vi "queue packet to transmit.vi"(8 "error in (no error)":errorcluster, 10 "Packet":string, 11 "data passing":T1) -> (0 "error out":errorcluster, 3 "data passing out":T1)   [LabVIEW 2016]
uses:
  data.ctl
  device/device.ctl
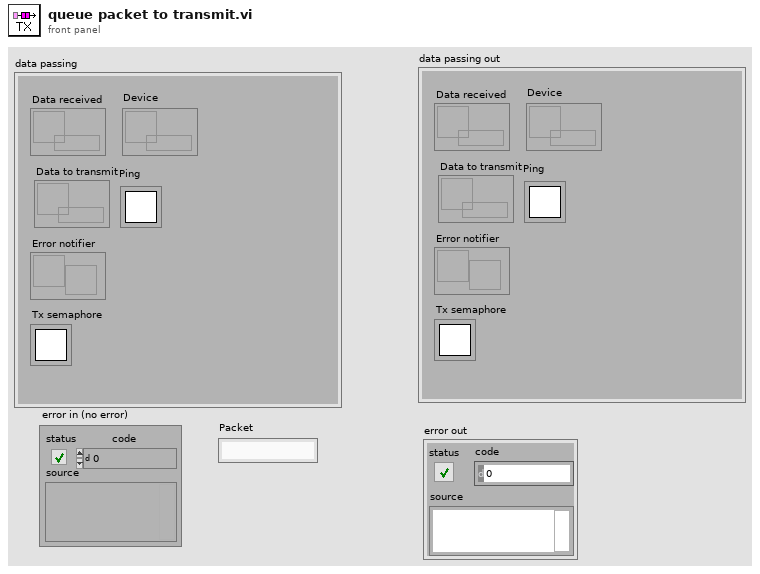
[diagram p1: front panel]
types:
  T1 = typedef "data.ctl" = cluster{"Data received":refnum<queue>, "Data to transmit":refnum<queue>, "Error notifier":refnum<notifier>, "Tx semaphore":T2, "Device":refnum<queue>, "Ping":T2}
  T2 = typedef "Semaphore RefNum" = refnum<k1>
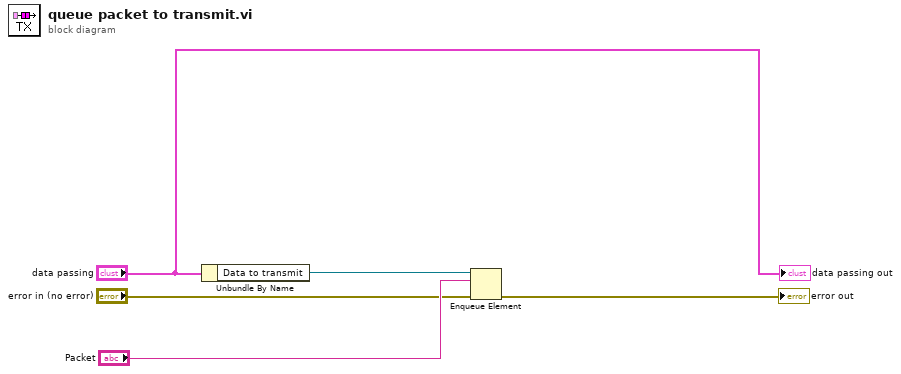
[diagram p0: block diagram]
diagram:
  n1 = Unbundle By Name("data passing") -> ("Data to transmit"=w4:refnum<queue>)
  n2 = Enqueue Element(queue=w4, element="Packet", error in (no error)="error in (no error)") -> (error out=→"error out":errorcluster)  [unwired: 1 in, 2 out]
  "data passing out" <- "data passing"
